vi "Connection Default.vi"(8 "error in":errorcluster, 11 "Acopian in":refnum<class "Acopian.lvclass">) -> (0 "error out":errorcluster, 3 "Acopian out":refnum<class "Acopian.lvclass">)   [LabVIEW 2019, in "Acopian.lvlib" / "Acopian.lvclass"]
uses:
  Library/Acopian.lvclass
  Library/Acopian.lvclass/Acopian.ctl
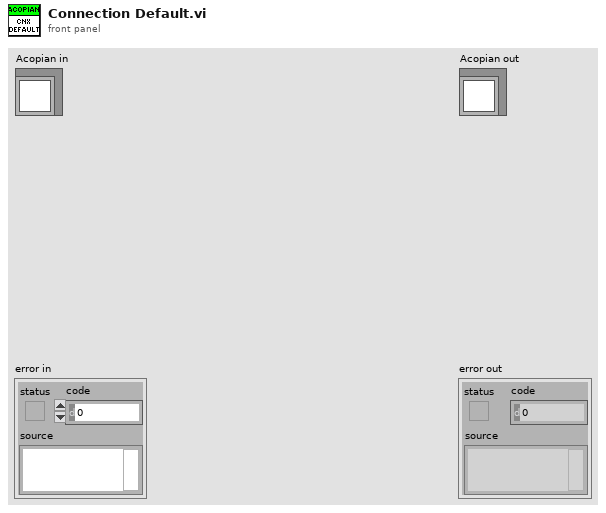
[diagram p1: front panel]
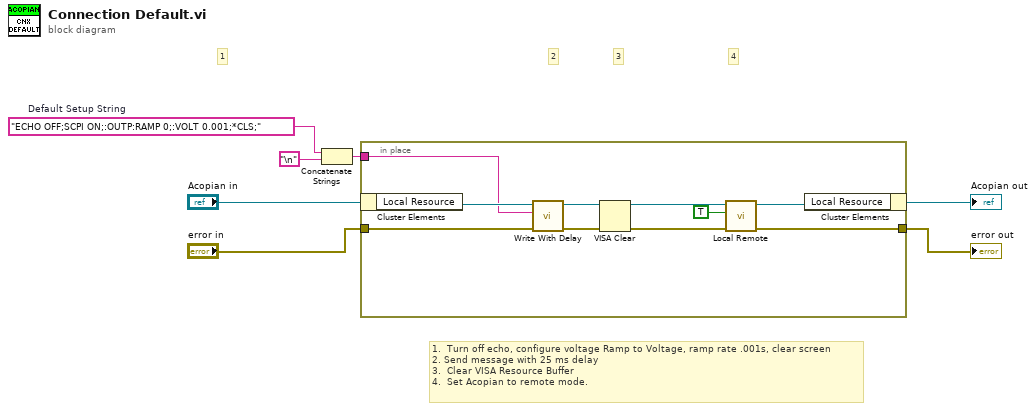
[diagram p0: block diagram]
diagram:
  w6 = "ECHO OFF;SCPI ON;:OUTP:RAMP 0;:VOLT 0.001;*CLS;"  # Default Setup String
  # "3"
  # "1.  Turn off echo, configure voltage Ramp to Voltage, ramp rate .001s, clear screen\n2. Send message with 25 ms delay\n3.  Clear VISA Resource Buffer\n4.  Set Acopian to remote mode."
  # "4"
  # "2"
  # "1"
  n1 = Concatenate Strings(w6, "\n") -> (w2:string)
  n2 = in-place {
    in-place-border: w2 -> [w16]
    in-place-border: "error in" -> [w14]
    in-place-border: [w13] -> w3
    n3 = in-place-cluster #1("Acopian in") -> ("Local Resource"=w17:refnum<visa-resource-name>)
    n4 = call "Write With Delay.vi"("error in"=w14, "write buffer"=w16, "VISA resource name"=w17) -> ("error out"=w8:errorcluster, "VISA resource name out"=w15:refnum<visa-resource-name>)  [unwired: 7 in]
    n5 = VISA Clear(VISA resource name=w15, error in (no error)=w8) -> (VISA resource name out=w11:refnum<visa-resource-name>, error out=w12:errorcluster)
    n6 = call "Local Remote.vi"("error in"=w12, "Remote (T: Remote)"=TRUE, "VISA resource name"=w11) -> ("error out"=w13:errorcluster, "VISA resource out"=w10:refnum<visa-resource-name>)  [unwired: 7 in]
    n7 = in-place-cluster #1("Local Resource"=w10) -> (→"Acopian out":refnum<class "Acopian.lvclass">)
  }
  "error out" <- w3
